vi "VIReadAnalog.vi"(2 "FPGA Interface Input":refnum<k20>) -> (1 "Analog Input":i16[](array[numeric]))   [LabVIEW 2012]
uses:
  <vilib>/Utility/error.llb/Error Cluster From Error Code.vi
  <vilib>/rvi/errors/niLvFpgaAdjustHostInterfaceError.vi
  <vilib>/rvi/interface/nirviReadWriteControl/nirviReadWriteControl.xnode
  NiFpgaLv.dll
  <vilib>/rvi/interface/Simulation/niFpgaSimulationCallBeginRW.vi
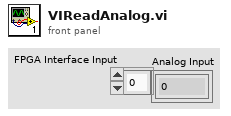
[diagram p1: front panel]
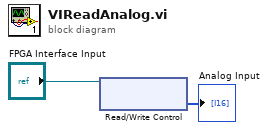
[diagram p0: block diagram]
diagram:
  n1 = xnode "Read/Write Control"("FPGA VI Reference In"="FPGA Interface Input") -> ("Analog Input"=→"Analog Input":i16[])  [unwired: 1 in, 2 out]
